vi "Clear Orphan.vi"(8 "error in (no error)":errorcluster, 11 "ArrayPanel in":refnum<class "ArrayPanel.lvclass">) -> (0 "error out":errorcluster, 3 "ArrayPanel out":refnum<class "ArrayPanel.lvclass">)   [LabVIEW 2020, in "OOPanel.lvlib" / "ArrayPanel.lvclass"]
uses:
  ArrayPanel.lvclass
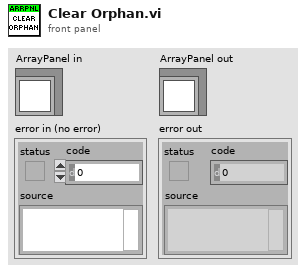
[diagram p1: front panel]
types:
  T1 = typedef "OOPanel.lvlib/ArrayPanel.lvclass/Ref Data.ctl" = cluster{"Orphan":bool}
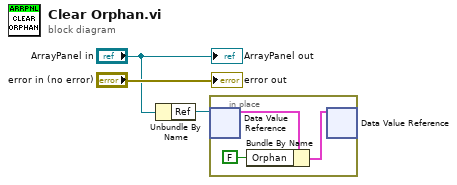
[diagram p0: block diagram]
diagram:
  n1 = Unbundle By Name("ArrayPanel in") -> ("Ref"=w2:refnum<data-value>)
  n2 = in-place {
    n3 = in-place-dvr #1(w2) -> (w6:T1)  [unwired: 1 out]
    n4 = Bundle By Name(cluster=w6, "Orphan"=FALSE) -> (w5:T1)
    n5 = in-place-dvr #1(w5) -> ()  [unwired: 2 out]
  }
  "error out" <- "error in (no error)"
  "ArrayPanel out" <- "ArrayPanel in"
